vi "SetClassQueueMessage.vi"(6 "QMessage":string, 8 "ErrorIn(No Error)":errorcluster caption="entrée d'erreur (pas d'erreur)", 9 "Data":variant, 10 "Menu déroulant":T1 items=["UpdateClassData", "UpdateMainClass", "UpdateDataBind", "ReInitDevice", "Custom", "ClosePan"], 11 "DefaultDev.lvclass":refnum<class "AFG3102C.lvclass">) -> (0 "sortie d'erreur":errorcluster, 3 "DefaultDev.lvclass Out":refnum<class "AFG3102C.lvclass">)   [LabVIEW 2019, in "AFG3102C.lvclass"]
uses:
  AFG3102C.lvclass
  BaseDevice/ClassQueueMess.ctl
  BaseDevice/BaseDevice.lvclass
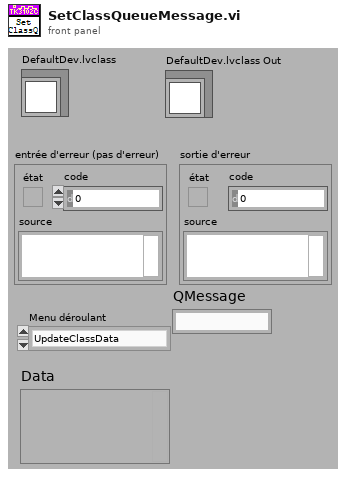
[diagram p1: front panel]
types:
  T1 = typedef "ClassQueueMess.ctl" = u16
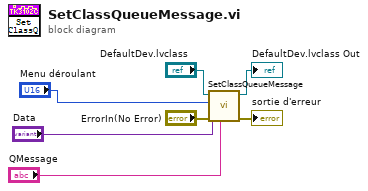
[diagram p0: block diagram]
diagram:
  n1 = call-parent "SetClassQueueMessage.vi"("QMessage"="QMessage", "ErrorIn(No Error)"="ErrorIn(No Error)", "Data"="Data", "Menu déroulant"="Menu déroulant", "BaseDevice.lvclass"="DefaultDev.lvclass") -> ("sortie d'erreur"=→"sortie d'erreur":errorcluster, "BaseDevice.lvclass Out"=→"DefaultDev.lvclass Out":refnum<class "AFG3102C.lvclass">)  [unwired: 5 in]
